vi "Periodic Tasks.vi"(8 "error in":errorcluster) -> ()   [LabVIEW 2014]
doc: "This VI runs in parallel to other tasks. It can contain as many user-defined periodic loops as you need. These can carry out PID or other sorts of timed response."
uses:
  <vilib>/Rock Robotics/WPI/Solenoid/WPI_SolenoidValue.ctl
  Robot Global Data.vi
  <vilib>/Rock Robotics/WPI/RobotDrive/WPI_RobotDriveGetSetRefNum.vi
  <vilib>/Rock Robotics/WPI/RobotDrive/WPI_RobotDriveMecanumDrive_Cartesian.vi
  <vilib>/Rock Robotics/WPI/Solenoid/WPI_SolenoidSetEnum.vi
  <vilib>/Rock Robotics/Network Tables/SD Read String.vi
  <vilib>/Rock Robotics/Network Tables/SD Read Boolean.vi
  <vilib>/Rock Robotics/Network Tables/SD Write Number.vi
  <vilib>/Rock Robotics/Network Tables/SD Write Boolean.vi
  navx-mxp_NEW/roborio/labview/navX-MXP Library/navX-MXP IMU.lvlib
panel:
  out "String":string
  out "Raw Yaw":dbl
  out "\"Field Centric\" Value":dbl
  out "North":dbl
  out "Level":dbl
  out "Wanted Level":dbl
  out "Left Switch":bool
  out "Right Switch":bool
  out "Bottom Switch":bool
  out "Top Switch":bool
  out "Adjusted Yaw":dbl
  out "Valid?":bool
  # "EDITED: 3/2/15"
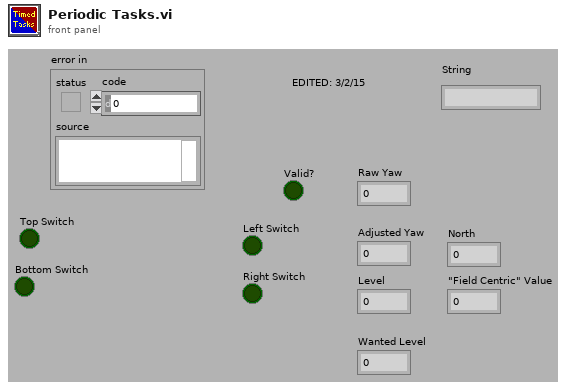
[diagram p1: front panel]
types:
  T1 = typedef "WPI_DigitalInputDevRef.ctl" = cluster{"DevStatus":errorcluster, "DIO Channel":T2, "Controller":T3}
  T2 = typedef "FPGA_DIOChannel.ctl" = enum8{"DIO 0", "DIO 1", "DIO 2", "DIO 3", "DIO 4", "DIO 5", "DIO 6", "DIO 7", "DIO 8", "DIO 9", "DIO MXP 0", "DIO MXP 1", "DIO MXP 2", "DIO MXP 3", "DIO MXP 4", "DIO MXP 5", "DIO MXP 6", "DIO MXP 7", "DIO MXP 8", "DIO MXP 9", "DIO MXP 10", "DIO MXP 11", "DIO MXP 12", "DIO MXP 13", "DIO MXP 14", "DIO MXP 15", "Invalid"}
  T3 = typedef "FPGA_TypedefDigitalModule.ctl" = enum16{"Controller 1"}
  T4 = typedef "navX-MXP IMU.lvlib/navX Device TypeDef.ctl" = cluster{"navX Interface Protocol":T5, "navX Interface Protocol TypeDefs":cluster{"SPIDevRef":T6, "I2CDevRef":T8}, "navX System Information":cluster{"Board Information":T10, "Status":T11, "Offsets":T15}, "navX Common Information":cluster{"Update Rate (4Hz-60Hz)":T16, "refnum name":string, "error":errorcluster}}
  T5 = typedef "navX-MXP IMU.lvlib/navX Interface Protocol.ctl" = enum16{"SPI", "I2C"}
  T6 = typedef "WPI_SPIDevRef.ctl" = cluster{"DevStatus":errorcluster, "Handle":i32, "Controller":T3, "SPI Bus":T7}
  T7 = typedef "spi_bus.ctl" = enum16{"SPI On-Board, CS0", "SPI On-Board, CS1", "SPI On-Board, CS2", "SPI On-Board, CS3", "SPI MXP", "Invalid"}
  T8 = typedef "WPI_I2CDevRef.ctl" = cluster{"DevStatus":errorcluster, "Controller":T3, "Device Address":u8, "Handle":i32, "I2C Bus":T9}
  T9 = typedef "i2c_bus.ctl" = enum16{"I2C On-Board", "I2C MXP", "Invalid"}
  T10 = typedef "navX-MXP IMU.lvlib/navX Board Information.ctl" = cluster{"WhoAmI (50 | 0x32)":u8, "Board Revision":u8, "Firmware Major Version":u8, "Firmware Minor Version":u8}
  T11 = typedef "navX-MXP IMU.lvlib/navX Status Data.ctl" = cluster{"Update Rate Hz":u8, "Accelerometer Full-Scale Range":u8, "Gyro Full-Scale Range":u16, "NAVX_OP_STATUS":T12, "NAVX_CAL_STATUS":T13, "NAVX_SELFTEST_STATUS":u8, "NAVX_SENSOR_STATUS":T14}
  T12 = typedef "navX-MXP IMU.lvlib/navX NAVX_OP_STATUS.ctl" = u8
  T13 = typedef "navX-MXP IMU.lvlib/navX NAVX_CAL_STATUS.ctl" = u8
  T14 = typedef "navX-MXP IMU.lvlib/navX NAVX_SENSOR_STATUS.ctl" = cluster{"MOVING":bool, "YAW_STABLE":bool, "MAG_DISTURBANCE":bool, "ALTITUDE_VALID":bool, "SEALEVEL_PRESS_SET":bool, "FUSED_HEADING_VALID":bool}
  T15 = typedef "navX-MXP IMU.lvlib/navX Offsets Data.ctl" = cluster{"Yaw":dbl, "Quat W":dbl, "Quat X":dbl, "Quat Y":dbl, "Quat Z":dbl}
  T16 = typedef "navX-MXP IMU.lvlib/navX Update Rate.ctl" = u8
  T17 = typedef "navX-MXP IMU.lvlib/navX YPRH Data.ctl" = cluster{"Yaw":dbl, "Pitch":dbl, "Roll":dbl, "Heading":dbl}
  T18 = typedef "WPI_RobotDriveDevRef.ctl" = cluster{"DevStatus":errorcluster, "Motors[]":T19[], "Square Inputs":bool, "Max Output":dbl}
  T19 = typedef "WPI_MotorControlDeviceRef.ctl" = cluster{"DeviceStatus":errorcluster, "Type":T20, "PWM":cluster{"Controller":T3, "PWM Channel":T21, "DeadBand":T22}, "CAN":cluster{"Device Number":u8, "Control Mode":T23, "Semaphore":T24, "Max Vout":dbl, "TalonSRX Control Mode":T25}, "Invert":bool, "TransformRef":T26, "InvTransformRef":T26}
  T20 = typedef "WPI_MotorControlType.ctl" = enum16{"PWM", "CAN", "CANTalonSRX"}
  T21 = typedef "FPGA_DIOPWMChannel.ctl" = enum8{"PWM 0", "PWM 1", "PWM 2", "PWM 3", "PWM 4", "PWM 5", "PWM 6", "PWM 7", "PWM 8", "PWM 9", "PWM MXP 0", "PWM MXP 1", "PWM MXP 2", "PWM MXP 3", "PWM MXP 4", "PWM MXP 5", "PWM MXP 6", "PWM MXP 7", "PWM MXP 8", "PWM MXP 9", "Invalid"}
  T22 = typedef "WPI_PWMDeadband.ctl" = cluster{"Name":string, "maxPositivePwm":i32, "minPositivePwm":i32, "centerPwm":i32, "maxNegativePwm":i32, "minNegativePwm":i32, "angularRange":u16}
  T23 = typedef "WPI_CANJaguar_ControlMode.ctl" = enum8{"Percent VBus", "Current", "Speed", "Position", "Voltage"}
  T24 = typedef "Semaphore RefNum" = refnum<k1>
  T25 = typedef "WPI_CANTalonSRX_APIControlMode.ctl" = enum8{"Percent VBus", "Speed", "Position", "Slave", "Unchanged / Invalid"}
  T26 = typedef "WPI_PWMTransform_ConPane.ctl" = refnum<vi>
  T27 = typedef "WPI_SolenoidDevRef.ctl" = cluster{"DevStatus":errorcluster, "Pneumatics Control Module":u8, "Forward Solenoid Channel":T28, "Reverse Solenoid Channel":T28}
  T28 = typedef "WPI_SolenoidChannel.ctl" = enum8{"Solenoid 0", "Solenoid 1", "Solenoid 2", "Solenoid 3", "Solenoid 4", "Solenoid 5", "Solenoid 6", "Solenoid 7", "Invalid"}
  T29 = typedef "WPI_SolenoidValue.ctl" = enum16{"Off", "On", "Forward", "Reverse"}
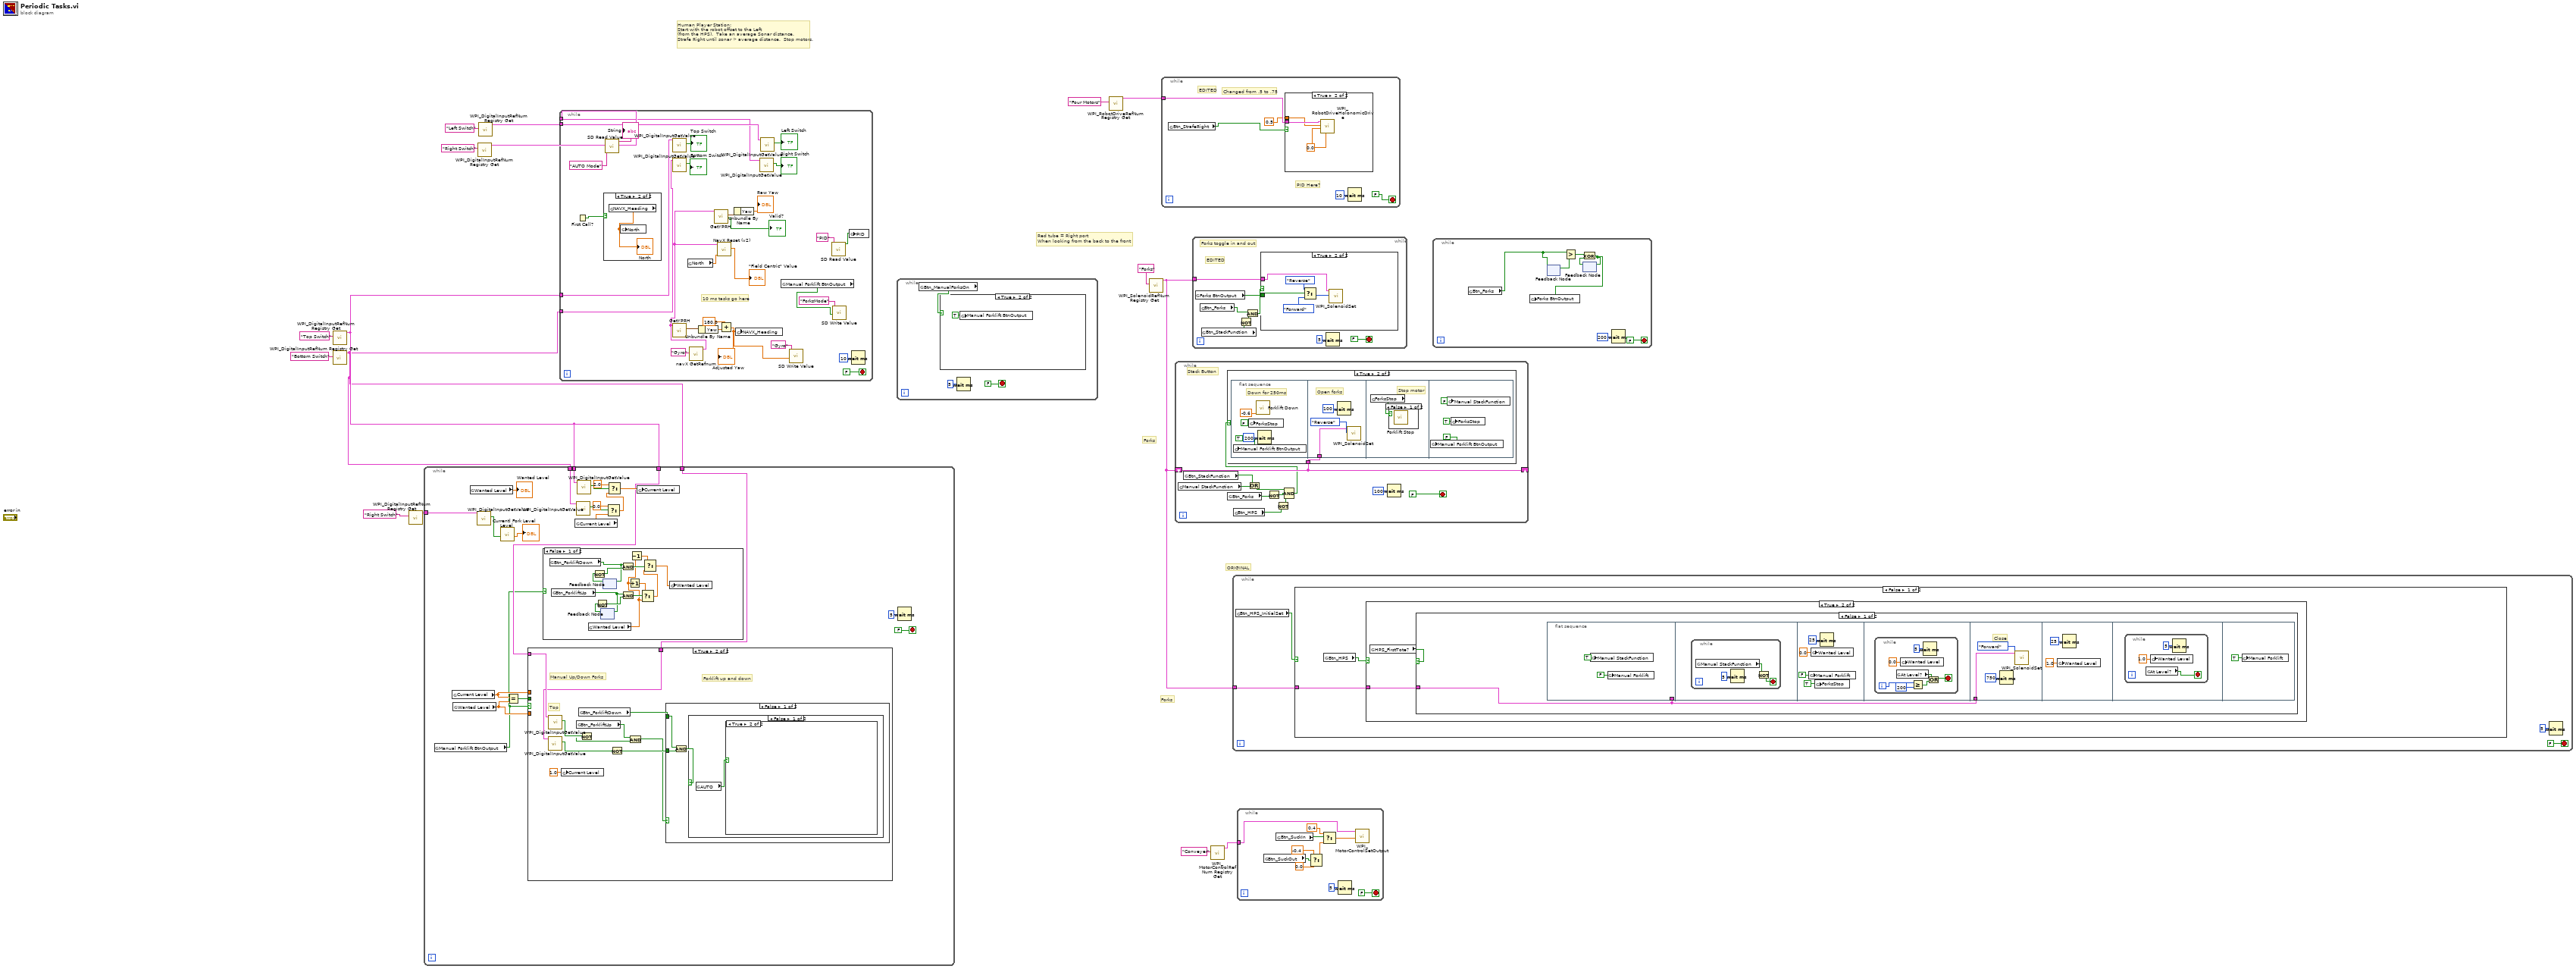
[diagram p0: block diagram]
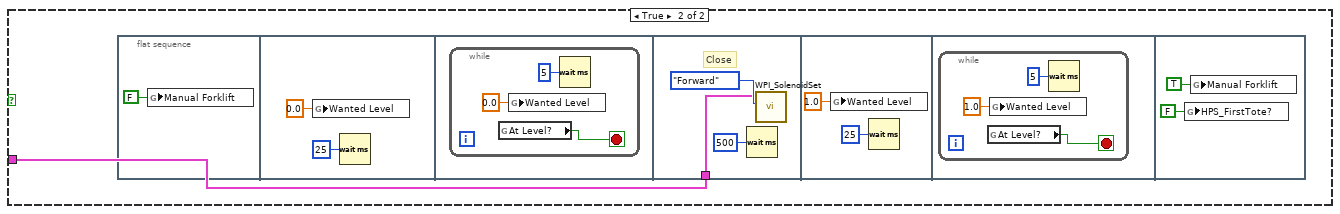
[diagram p3: hidden frame]
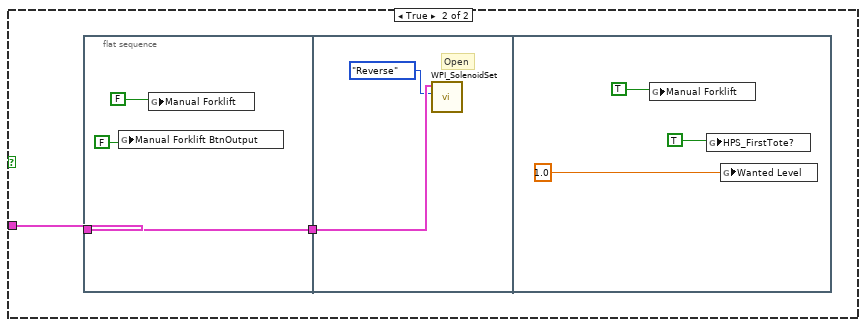
[diagram p4: hidden frame]
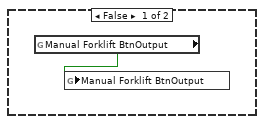
[diagram p6: hidden frame]
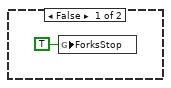
[diagram p7: hidden frame]
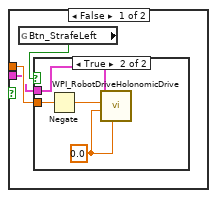
[diagram p10: hidden frame]
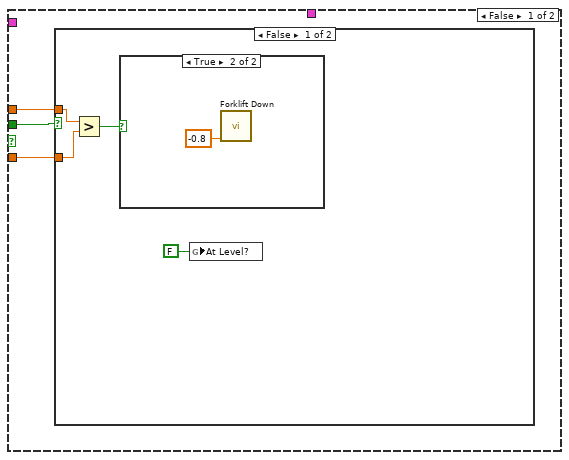
[diagram p13: hidden frame]
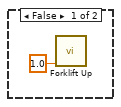
[diagram p14: hidden frame]
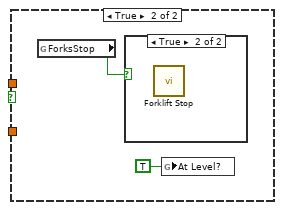
[diagram p15: hidden frame]
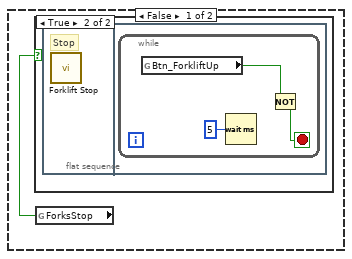
[diagram p17: hidden frame]
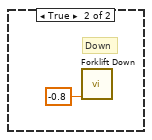
[diagram p19: hidden frame]
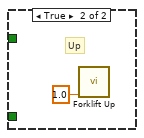
[diagram p20: hidden frame]
diagram:
  # "ORIGINAL"
  # "Forks"
  # "Forks"
  # "Human Player Station:\nStart with the robot offset to the Left\n(from the HPS).  Take an average Sonar distance.\nStrafe Right until sonar > average distance.  Stop motors."
  # "Red tube = Right port\nWhen looking from the back to the front"
  n1 = call <vilib>:"WPI_DigitalInputRefNum Registry Get.vi"("refnum name"="Bottom Switch") -> ("DigitalInputDevRef"=w3:T1)  [unwired: 9 in, 1 out]
  n2 = call <vilib>:"WPI_DigitalInputRefNum Registry Get.vi"("refnum name"="Top Switch") -> ("DigitalInputDevRef"=w4:T1)  [unwired: 9 in, 1 out]
  n3 = call <vilib>:"WPI_DigitalInputRefNum Registry Get.vi"("refnum name"="Right Switch") -> ("DigitalInputDevRef"=w12:T1)  [unwired: 9 in, 1 out]
  n4 = while {
    tunnel: w4 -> [w28]
    tunnel: w3 -> [w27]
    tunnel: w12 -> [w25]
    tunnel: w4 -> [w20]
    tunnel: w3 -> [w19]
    stop <- FALSE stop-if-true
    n5 = global read "Robot Global Data.vi" "Manual Forklift BtnOutput"() -> (w17:bool)
    n6 = global read "Robot Global Data.vi" "Current Level"() -> (w22:dbl)
    n7 = global read "Robot Global Data.vi" "Wanted Level"() -> (w21:dbl)
    n8 = global read "Robot Global Data.vi" "Wanted Level"() -> (→"Wanted Level":dbl)
    n9 = call <vilib>:"WPI_DigitalInputGetValue.vi"("DigitalInputDevRef"=w25) -> ("Value"=w18:bool)  [unwired: 8 in, 2 out]
    n10 = call "Currentl Fork Level.vi"("Right"=w18) -> ("Level"=→"Level":dbl)  [unwired: 10 in]
    n11 = Equal?(x=w22, y=w21) -> (x = y?=w23:bool)
    n12 = case shown="True" w17 {
      tunnel: w23 -> [w53 _]
      tunnel: w22 -> [w52 _]
      tunnel: w21 -> [w51 _]
      tunnel: w20 -> [_ w64]
      tunnel: w19 -> [_ w63]
      frame False {
        n13 = case shown="False" w53 {
          tunnel: w52 -> [w55 _]
          tunnel: w51 -> [w54 _]
          frame False {
            n14 = Greater?(x=w55, y=w54) -> (0:w57:bool)
            n15 = case shown="True" w57 {
              frame False {
                n16 = call "Forklift Up.vi"("Forklift Up Power"=1.0) -> ()  [unwired: 11 in]
              }
              frame True {
                n17 = call "Forklift Down.vi"("Forklift Down Speed"=-0.8) -> ()  [unwired: 11 in]
              }
            }
            n18 = global write "Robot Global Data.vi" "At Level?"(FALSE ("ForksStop")) -> ()
          }
          frame True {
            n19 = global read "Robot Global Data.vi" "ForksStop"() -> (w61:bool)
            n20 = case shown="True" w61 {
              frame False {
              }
              frame True {
                n21 = call "Forklift Stop.vi"() -> ()  [unwired: 12 in]
              }
            }
            n22 = global write "Robot Global Data.vi" "At Level?"(TRUE ("ForksStop")) -> ()
          }
        }
      }
      frame True {
        # "Top"
        # "Forklift up and down"
        # "Manual Up/Down Forks"
        n23 = call <vilib>:"WPI_DigitalInputGetValue.vi"("DigitalInputDevRef"=w63) -> ("Value"=w70:bool)  [unwired: 8 in, 2 out]
        n24 = call <vilib>:"WPI_DigitalInputGetValue.vi"("DigitalInputDevRef"=w64) -> ("Value"=w71:bool)  [unwired: 8 in, 2 out]
        n25 = global write "Robot Global Data.vi" "Current Level"(1.0 ("Current Level")) -> ()
        n26 = global read "Robot Global Data.vi" "Btn_ForkliftUp"() -> (w67:bool)
        n27 = global read "Robot Global Data.vi" "Btn_ForkliftDown"() -> (w69:bool)
        n28 = Not(x=w71) -> (.not. x?=w66:bool)
        n29 = Not(x=w70) -> (.not. x?=w68:bool)
        n30 = And(x=w67, y=w66) -> (x .and. y?=w65:bool)
        n31 = case shown="False" w65 {
          tunnel: w69 -> [w72 _]
          tunnel: w68 -> [w73 _]
          frame False {
            n32 = And(x=w72, y=w73) -> (x .and. y?=w74:bool)
            n33 = case shown="False" w74 {
              frame False {
                n34 = global read "Robot Global Data.vi" "AUTO"() -> (w75:bool)
                n35 = case shown="True" w75 {
                  frame False {
                    n36 = global read "Robot Global Data.vi" "ForksStop"() -> (w76:bool)
                    n37 = case shown="True" w76 {
                      frame False {
                      }
                      frame True {
                        n38 = flat-sequence {
                          frame #0 {
                            # "Stop"
                            n39 = call "Forklift Stop.vi"() -> ()  [unwired: 12 in]
                          }
                          frame #1 {
                            n40 = while {
                              stop <- w77 stop-if-true
                              n41 = global read "Robot Global Data.vi" "Btn_ForkliftUp"() -> (w78:bool)
                              n42 = Wait (ms)(milliseconds to wait=u32 5) -> ()  [unwired: 1 out]
                              n43 = Not(x=w78) -> (.not. x?=w77:bool)
                            }
                          }
                        }
                      }
                    }
                  }
                  frame True {
                  }
                }
              }
              frame True {
                # "Down"
                n44 = call "Forklift Down.vi"("Forklift Down Speed"=-0.8) -> ()  [unwired: 11 in]
              }
            }
          }
          frame True {
            # "Up"
            n45 = call "Forklift Up.vi"("Forklift Up Power"=1.0) -> ()  [unwired: 11 in]
          }
        }
      }
    }
    n46 = case shown="False" w17 {
      frame False {
        n47 = global read "Robot Global Data.vi" "Btn_ForkliftDown"() -> (w45:bool)
        n48 = global read "Robot Global Data.vi" "Btn_ForkliftUp"() -> (w49:bool)
        n49 = global read "Robot Global Data.vi" "Wanted Level"() -> (w38:dbl)
        n50 = feedback #1() -> (w48:bool)  [unwired: 1 in]
        n51 = Not(x=w48) -> (.not. x?=w50:bool)
        n52 = feedback-in #1(w49) -> ()
        n53 = feedback #2() -> (w46:bool)  [unwired: 1 in]
        n54 = Not(x=w46) -> (.not. x?=w47:bool)
        n55 = feedback-in #2(w45) -> ()
        n56 = And(x=w45, y=w47) -> (x .and. y?=w44:bool)
        n57 = And(x=w49, y=w50) -> (x .and. y?=w43:bool)
        n58 = Increment(x=w38) -> (x+1=w41:dbl)
        n59 = Decrement(x=w38) -> (x-1=w39:dbl)
        n60 = Select(t=w41, s=w43, f=w38) -> (s? t:f=w42:dbl)
        n61 = Select(t=w39, s=w44, f=w42) -> (s? t:f=w40:dbl)
        n62 = global write "Robot Global Data.vi" "Wanted Level"(w40) -> ()
      }
      frame True {
      }
    }
    n63 = global read "Robot Global Data.vi" "Current Level"() -> (w35:dbl)
    n64 = call <vilib>:"WPI_DigitalInputGetValue.vi"("DigitalInputDevRef"=w27) -> ("Value"=w30:bool)  [unwired: 8 in, 2 out]
    n65 = call <vilib>:"WPI_DigitalInputGetValue.vi"("DigitalInputDevRef"=w28) -> ("Value"=w29:bool)  [unwired: 8 in, 2 out]
    n66 = Select(t=0.0, s=w30, f=w35) -> (s? t:f=w34:dbl)
    n67 = Select(t=2.0, s=w29, f=w34) -> (s? t:f=w33:dbl)
    n68 = global write "Robot Global Data.vi" "Current Level"(w33) -> ()
    n69 = Wait (ms)(milliseconds to wait=u32 5) -> ()  [unwired: 1 out]
  }
  n70 = call <vilib>:"WPI_DigitalInputRefNum Registry Get.vi"("refnum name"="Right Switch") -> ("DigitalInputDevRef"=w5:T1)  [unwired: 9 in, 1 out]
  n71 = call <vilib>:"WPI_DigitalInputRefNum Registry Get.vi"("refnum name"="Left Switch") -> ("DigitalInputDevRef"=w6:T1)  [unwired: 9 in, 1 out]
  n72 = while {
    tunnel: w4 -> [w108]
    tunnel: w3 -> [w107]
    tunnel: w6 -> [w102]
    tunnel: w5 -> [w101]
    stop <- FALSE stop-if-true
    # "10 ms tasks go here"
    n73 = First Call?() -> (First Call?: T/F=w91:bool)
    n74 = case shown="True" w91 {
      frame False {
      }
      frame True {
        n75 = global read "Robot Global Data.vi" "NAVX_Heading"() -> (w111:dbl)
        "North" <- w111
        n76 = global write "Robot Global Data.vi" "North"(w111) -> ()
      }
    }
    n77 = call-poly <vilib>:"SD Read Value.vi"("Name"="AUTO Mode") -> ("String"=→"String":string)  [unwired: 8 in, 2 out]
    n78 = call <vilib>:"WPI_DigitalInputGetValue.vi"("DigitalInputDevRef"=w107) -> ("Value"=→"Bottom Switch":bool)  [unwired: 8 in, 2 out]
    n79 = call <vilib>:"WPI_DigitalInputGetValue.vi"("DigitalInputDevRef"=w108) -> ("Value"=→"Top Switch":bool)  [unwired: 8 in, 2 out]
    n80 = global read "Robot Global Data.vi" "North"() -> (w90:dbl)
    n81 = call "navX GetRefnum.vi"("refnum name"="Gyro") -> ("navX Device TypeDef"=w92:T4)  [unwired: 9 in, 1 out]
    n82 = call "GetYPRH.vi"("navX Device TypeDef"=w92) -> ("YPRH"=w100:T17)  [unwired: 8 in, 2 out]
    n83 = Unbundle By Name(w100) -> ("Yaw"=w99:dbl)
    n84 = call "GetYPRH.vi"("navX Device TypeDef"=w92) -> ("Valid?"=→"Valid?":bool, "YPRH"=w95:T17)  [unwired: 8 in, 1 out]
    n85 = call "NavX Reset (v2).vi"("North In"=w90, "navX Device TypeDef"=w92) -> ("Output Angle"=→"\"Field Centric\" Value":dbl)  [unwired: 9 in]
    n86 = Add(x=180.0, y=w99) -> (x+y=w83:dbl)
    "Adjusted Yaw" <- w83
    n87 = Unbundle By Name(w95) -> ("Yaw"=→"Raw Yaw":dbl)
    n88 = global write "Robot Global Data.vi" "NAVX_Heading"(w83) -> ()
    n89 = call <vilib>:"WPI_DigitalInputGetValue.vi"("DigitalInputDevRef"=w101) -> ("Value"=→"Right Switch":bool)  [unwired: 8 in, 2 out]
    n90 = call <vilib>:"WPI_DigitalInputGetValue.vi"("DigitalInputDevRef"=w102) -> ("Value"=→"Left Switch":bool)  [unwired: 8 in, 2 out]
    n91 = global read "Robot Global Data.vi" "Manual Forklift BtnOutput"() -> (w86:bool)
    n92 = call-poly <vilib>:"SD Write Value.vi"("Numeric"=w83, "Name"="Gyro") -> ()  [unwired: 8 in, 2 out]
    n93 = call-poly <vilib>:"SD Read Value.vi"("Name"="PID") -> ("Boolean"=w84:bool)  [unwired: 8 in, 2 out]
    n94 = call-poly <vilib>:"SD Write Value.vi"("Boolean"=w86, "Name"="ForksMode") -> ()  [unwired: 8 in, 2 out]
    n95 = global write "Robot Global Data.vi" "PID"(w84) -> ()
    n96 = Wait (ms)(milliseconds to wait=u32 10) -> ()  [unwired: 1 out]
  }
  n97 = while {
    stop <- FALSE stop-if-true
    n98 = global read "Robot Global Data.vi" "Btn_ManualForksOn"() -> (w112:bool)
    n99 = case shown="True" w112 {
      frame False {
        n100 = global read "Robot Global Data.vi" "Manual Forklift BtnOutput"() -> (w115:bool)
        n101 = global write "Robot Global Data.vi" "Manual Forklift BtnOutput"(w115) -> ()
      }
      frame True {
        n102 = global write "Robot Global Data.vi" "Manual Forklift BtnOutput"(TRUE ("Btn_ManualDriveToggle")) -> ()
      }
    }
    n103 = Wait (ms)(milliseconds to wait=u32 5) -> ()  [unwired: 1 out]
  }
  n104 = call <vilib>:"WPI_RobotDriveRefNum Registry Get.vi"("refnum name"="Four Motors") -> ("RobotDriveDevRef"=w10:T18)  [unwired: 9 in, 1 out]
  n105 = call <vilib>:"WPI_SolenoidRefNum Registry Get.vi"("refnum name"="Forks") -> ("SolenoidDevRef"=w14:T27)  [unwired: 9 in, 1 out]
  n106 = while {
    tunnel: w10 -> [w119]
    stop <- FALSE stop-if-true
    # "Changed from .5 to .75"
    # "EDITED"
    # "PID Here?"
    n107 = global read "Robot Global Data.vi" "Btn_StrafeRight"() -> (w117:bool)
    n108 = case shown="True" w117 {
      tunnel: w119 -> [w122 w131]
      tunnel: 0.5 ("t") -> [w123 w130]
      frame False {
        n109 = global read "Robot Global Data.vi" "Btn_StrafeLeft"() -> (w124:bool)
        n110 = case shown="True" w124 {
          tunnel: w123 -> [_ w128]
          tunnel: w122 -> [_ w126]
          frame False {
          }
          frame True {
            w125 = 0.0 ("Rotation")
            n111 = Negate(x=w128) -> (-x=w127:dbl)
            n112 = call-poly <vilib>:"WPI_RobotDriveHolonomicDrive.vi"("Rotation"=w125, "Y"=w125, "X"=w127, "RobotDriveDevRef"=w126) -> ()  [unwired: 5 in, 3 out]
          }
        }
      }
      frame True {
        w129 = 0.0 ("Rotation")
        n113 = call-poly <vilib>:"WPI_RobotDriveHolonomicDrive.vi"("Rotation"=w129, "Y"=w129, "X"=w130, "RobotDriveDevRef"=w131) -> ()  [unwired: 5 in, 3 out]
      }
    }
    n114 = Wait (ms)(milliseconds to wait=u32 10) -> ()  [unwired: 1 out]
  }
  n115 = while {
    shift-right: [w140] -> _
    shift-left: w14 -> [w140]
    stop <- FALSE stop-if-true
    # "Stack Button"
    n116 = global read "Robot Global Data.vi" "Manual StackFunction"() -> (w132:bool)
    n117 = global read "Robot Global Data.vi" "Btn_StackFunction"() -> (w139:bool)
    n118 = global read "Robot Global Data.vi" "Btn_Forks"() -> (w138:bool)
    n119 = global read "Robot Global Data.vi" "Btn_HPS"() -> (w135:bool)
    n120 = Or(x=w139, y=w132) -> (x .or. y?=w133:bool)
    n121 = Not(x=w138) -> (.not. x?=w137:bool)
    n122 = Not(x=w135) -> (.not. x?=w134:bool)
    n123 = Compound Arithmetic op=AND(w133, w137, w134) -> (w136:bool)
    n124 = case shown="True" w136 {
      tunnel: w140 -> [_ w144]
      frame False {
        n125 = global write "Robot Global Data.vi" "ForksStop"(TRUE ("ForksStop")) -> ()
      }
      frame True {
        n126 = flat-sequence {
          tunnel: w144 -> [w149]
          frame #0 {
            # "Down for 250ms"
            n127 = global write "Robot Global Data.vi" "Manual Forklift BtnOutput"(TRUE ("Manual Forklift")) -> ()
            n128 = global write "Robot Global Data.vi" "ForksStop"(FALSE ("ForksStop")) -> ()
            n129 = call "Forklift Down.vi"("Forklift Down Speed"=-0.6) -> ()  [unwired: 11 in]
            n130 = Wait (ms)(milliseconds to wait=u32 200) -> ()  [unwired: 1 out]
          }
          frame #1 {
            # "Open forks"
            n131 = Wait (ms)(milliseconds to wait=u32 100) -> ()  [unwired: 1 out]
            n132 = call-poly <vilib>:"WPI_SolenoidSet.vi"("Value"=WPI_SolenoidValue."Reverse", "SolenoidDevRef"=w149) -> ()  [unwired: 8 in, 2 out]
          }
          frame #2 {
            # "Stop motor"
            n133 = global read "Robot Global Data.vi" "ForksStop"() -> (w152:bool)
            n134 = case shown="False" w152 {
              frame False {
                n135 = call "Forklift Stop.vi"() -> ()  [unwired: 12 in]
              }
              frame True {
              }
            }
          }
          frame #3 {
            n136 = global write "Robot Global Data.vi" "Manual Forklift BtnOutput"(FALSE ("ForksStop")) -> ()
            n137 = global write "Robot Global Data.vi" "Manual StackFunction"(FALSE ("Btn_StackFunction")) -> ()
            n138 = global write "Robot Global Data.vi" "ForksStop"(TRUE ("ForksStop")) -> ()
          }
        }
      }
    }
    n139 = Wait (ms)(milliseconds to wait=u32 100) -> ()  [unwired: 1 out]
  }
  n140 = while {
    tunnel: w14 -> [w156]
    stop <- FALSE stop-if-true
    # "EDITED"
    # "Forks toggle in and out"
    n141 = global read "Robot Global Data.vi" "Forks BtnOutput"() -> (w158:bool)
    n142 = global read "Robot Global Data.vi" "Btn_Forks"() -> (w157:bool)
    n143 = global read "Robot Global Data.vi" "Btn_StackFunction"() -> (w161:bool)
    n144 = Not(x=w161) -> (.not. x?=w160:bool)
    n145 = And(x=w157, y=w160) -> (x .and. y?=w159:bool)
    n146 = case shown="True" w159 {
      tunnel: w156 -> [_ w164]
      tunnel: w158 -> [_ w167]
      frame False {
      }
      frame True {
        n147 = Select(t=WPI_SolenoidValue."Reverse", s=w167, f=WPI_SolenoidValue."Forward" ("Value")) -> (s? t:f=w166:T29)
        n148 = call-poly <vilib>:"WPI_SolenoidSet.vi"("Value"=w166, "SolenoidDevRef"=w164) -> ()  [unwired: 8 in, 2 out]
      }
    }
    n149 = Wait (ms)(milliseconds to wait=u32 5) -> ()  [unwired: 1 out]
  }
  n150 = call <vilib>:"WPI_MotorControlRefNum Registry Get.vi"("refnum name"="Conveyer") -> ("MotorControlDevRef"=w1:T19)  [unwired: 9 in, 1 out]
  n151 = while {
    tunnel: w14 -> [w169]
    stop <- FALSE stop-if-true
    n152 = global read "Robot Global Data.vi" "Btn_HPS_InitialSet"() -> (w170:bool)
    n153 = case shown="False" w170 {
      tunnel: w169 -> [w173 w221]
      frame False {
        n154 = global read "Robot Global Data.vi" "Btn_HPS"() -> (w174:bool)
        n155 = case shown="True" w174 {
          tunnel: w173 -> [_ w175]
          frame False {
          }
          frame True {
            n156 = global read "Robot Global Data.vi" "HPS_FirstTote?"() -> (w176:bool)
            n157 = case shown="False" w176 {
              tunnel: w175 -> [w177 w203]
              frame False {
                n158 = flat-sequence {
                  tunnel: w177 -> [_]
                  tunnel: w177 -> [w194]
                  frame #0 {
                    n159 = global write "Robot Global Data.vi" "Manual StackFunction"(TRUE ("Btn_StackFunction")) -> ()
                    n160 = global write "Robot Global Data.vi" "Manual Forklift"(FALSE ("HPS_FirstTote?")) -> ()
                  }
                  frame #1 {
                    n161 = while {
                      stop <- w180 stop-if-true
                      n162 = global read "Robot Global Data.vi" "Manual StackFunction"() -> (w182:bool)
                      n163 = Wait (ms)(milliseconds to wait=u32 5) -> ()  [unwired: 1 out]
                      n164 = Not(x=w182) -> (.not. x?=w180:bool)
                    }
                  }
                  frame #2 {
                    n165 = global write "Robot Global Data.vi" "Manual Forklift"(FALSE ("HPS_FirstTote?")) -> ()
                    n166 = global write "Robot Global Data.vi" "Wanted Level"(0.0 ("Wanted Level")) -> ()
                    n167 = global write "Robot Global Data.vi" "ForksStop"(TRUE ("ForksStop")) -> ()
                    n168 = Wait (ms)(milliseconds to wait=u32 25) -> ()  [unwired: 1 out]
                  }
                  frame #3 {
                    n169 = while {
                      i -> [w190]
                      stop <- w188 stop-if-true
                      n170 = global read "Robot Global Data.vi" "At Level?"() -> (w193:bool)
                      n171 = global write "Robot Global Data.vi" "Wanted Level"(0.0 ("Wanted Level")) -> ()
                      n172 = Greater Or Equal?(x=w190, y=200) -> (x >= y?=w187:bool)
                      n173 = Wait (ms)(milliseconds to wait=u32 5) -> ()  [unwired: 1 out]
                      n174 = Or(x=w193, y=w187) -> (x .or. y?=w188:bool)
                    }
                  }
                  frame #4 {
                    # "Close"
                    n175 = Wait (ms)(milliseconds to wait=u32 750) -> ()  [unwired: 1 out]
                    n176 = call-poly <vilib>:"WPI_SolenoidSet.vi"("Value"=WPI_SolenoidValue."Forward", "SolenoidDevRef"=w194) -> ()  [unwired: 8 in, 2 out]
                  }
                  frame #5 {
                    n177 = global write "Robot Global Data.vi" "Wanted Level"(1.0 ("Wanted Level")) -> ()
                    n178 = Wait (ms)(milliseconds to wait=u32 25) -> ()  [unwired: 1 out]
                  }
                  frame #6 {
                    n179 = while {
                      stop <- w201 stop-if-true
                      n180 = global read "Robot Global Data.vi" "At Level?"() -> (w201:bool)
                      n181 = global write "Robot Global Data.vi" "Wanted Level"(1.0 ("Wanted Level")) -> ()
                      n182 = Wait (ms)(milliseconds to wait=u32 5) -> ()  [unwired: 1 out]
                    }
                  }
                  frame #7 {
                    n183 = global write "Robot Global Data.vi" "Manual Forklift"(TRUE ("HPS_FirstTote?")) -> ()
                  }
                }
              }
              frame True {
                n184 = flat-sequence {
                  tunnel: w203 -> [w211]
                  frame #0 {
                    n185 = global write "Robot Global Data.vi" "Manual Forklift"(FALSE ("Manual Forklift")) -> ()
                  }
                  frame #1 {
                    n186 = global write "Robot Global Data.vi" "Wanted Level"(0.0 ("Wanted Level")) -> ()
                    n187 = Wait (ms)(milliseconds to wait=u32 25) -> ()  [unwired: 1 out]
                  }
                  frame #2 {
                    n188 = while {
                      stop <- w209 stop-if-true
                      n189 = global read "Robot Global Data.vi" "At Level?"() -> (w209:bool)
                      n190 = global write "Robot Global Data.vi" "Wanted Level"(0.0 ("Wanted Level")) -> ()
                      n191 = Wait (ms)(milliseconds to wait=u32 5) -> ()  [unwired: 1 out]
                    }
                  }
                  frame #3 {
                    # "Close"
                    n192 = Wait (ms)(milliseconds to wait=u32 500) -> ()  [unwired: 1 out]
                    n193 = call-poly <vilib>:"WPI_SolenoidSet.vi"("Value"=WPI_SolenoidValue."Forward", "SolenoidDevRef"=w211) -> ()  [unwired: 8 in, 2 out]
                  }
                  frame #4 {
                    n194 = global write "Robot Global Data.vi" "Wanted Level"(1.0 ("Wanted Level")) -> ()
                    n195 = Wait (ms)(milliseconds to wait=u32 25) -> ()  [unwired: 1 out]
                  }
                  frame #5 {
                    n196 = while {
                      stop <- w217 stop-if-true
                      n197 = global read "Robot Global Data.vi" "At Level?"() -> (w217:bool)
                      n198 = global write "Robot Global Data.vi" "Wanted Level"(1.0 ("Wanted Level")) -> ()
                      n199 = Wait (ms)(milliseconds to wait=u32 5) -> ()  [unwired: 1 out]
                    }
                  }
                  frame #6 {
                    n200 = global write "Robot Global Data.vi" "HPS_FirstTote?"(FALSE ("HPS_FirstTote?")) -> ()
                    n201 = global write "Robot Global Data.vi" "Manual Forklift"(TRUE ("Manual Forklift")) -> ()
                  }
                }
              }
            }
          }
        }
      }
      frame True {
        n202 = flat-sequence {
          tunnel: w221 -> [w224]
          tunnel: [w224] -> w220
          tunnel: w220 -> [w226]
          frame #0 {
            n203 = global write "Robot Global Data.vi" "Manual Forklift BtnOutput"(FALSE ("HPS_FirstTote?")) -> ()
            n204 = global write "Robot Global Data.vi" "Manual Forklift"(FALSE ("HPS_FirstTote?")) -> ()
          }
          frame #1 {
            # "Open"
            n205 = call-poly <vilib>:"WPI_SolenoidSet.vi"("Value"=WPI_SolenoidValue."Reverse", "SolenoidDevRef"=w226) -> ()  [unwired: 8 in, 2 out]
          }
          frame #2 {
            n206 = global write "Robot Global Data.vi" "Manual Forklift"(TRUE ("HPS_FirstTote?")) -> ()
            n207 = global write "Robot Global Data.vi" "HPS_FirstTote?"(TRUE ("HPS_FirstTote?")) -> ()
            n208 = global write "Robot Global Data.vi" "Wanted Level"(1.0 ("Wanted Level")) -> ()
          }
        }
      }
    }
    n209 = Wait (ms)(milliseconds to wait=u32 5) -> ()  [unwired: 1 out]
  }
  n210 = while {
    tunnel: w1 -> [w230]
    stop <- FALSE stop-if-true
    n211 = global read "Robot Global Data.vi" "Btn_SuckOut"() -> (w237:bool)
    n212 = global read "Robot Global Data.vi" "Btn_SuckIn"() -> (w239:bool)
    n213 = Select(t=-0.4, s=w237, f=0.0) -> (s? t:f=w238:dbl)
    n214 = Select(t=0.4, s=w239, f=w238) -> (s? t:f=w233:dbl)
    n215 = Wait (ms)(milliseconds to wait=u32 5) -> ()  [unwired: 1 out]
    n216 = call <vilib>:"WPI_MotorControlSetOutput.vi"("Output"=w233, "MotorControlDevRef"=w230) -> ()  [unwired: 7 in, 3 out]
  }
  n217 = while {
    stop <- FALSE stop-if-true
    n218 = global read "Robot Global Data.vi" "Btn_Forks"() -> (w241:bool)
    n219 = feedback #3() -> (w244:bool)  [unwired: 1 out]
    n220 = feedback-in #3(w241) -> ()
    n221 = Greater?(x=w241, y=w244) -> (0:w243:bool)
    n222 = feedback #4() -> (w242:bool)  [unwired: 1 out]
    n223 = Exclusive Or(1:w242, 2:w243) -> (0:w240:bool)
    n224 = global write "Robot Global Data.vi" "Forks BtnOutput"(w240) -> ()
    n225 = feedback-in #4(w240) -> ()
    n226 = Wait (ms)(milliseconds to wait=u32 200) -> ()  [unwired: 1 out]
  }
